vi "Init.vi"   [LabVIEW 2009, in "IDW.lvlib"]
doc: "Initializes an I2C waveform. Timing parameters are coerced to edges at the given sample rate. The coerced values are output from the VI.\n\nThis VI is polymorphic. In the <b>Preallocated</b> instance (default), buffers are preallocated in memory for the I2C waveform generation operations. The buffer size must be input. In the <b>No allocation</b> instance, no buffers are allocated, and each operation on the waveform manages its own buffer every time it is called."
uses:
  IDW.lvlib
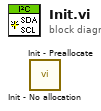
[diagram p0: block diagram]
diagram:
  n1 = call "Init - No allocation.vi"() -> ()  [unwired: 8 in, 4 out]
  n2 = call "Init - Preallocate.vi"() -> ()  [unwired: 8 in, 4 out]
